vi "Mandelbrot_LabVIEW.vi"() -> ()   [LabVIEW 2020]
uses:
  <vilib>/Analysis/1siggen.llb/Ramp Pattern by Samples.vi
  5424d61b-997c-4bc6-ad91-23142d452257.vi
  acdee1ab-0b82-4047-983d-88c3d57dfc2c.vi
  <vilib>/Analysis/NI_AALBase.lvlib
panel:
  out "Device":string="Intel(R) Core(TM) i7-8700K"
  out "Current Frame":i32=223
  out "Time Elapsed":dbl=579.0 format="%#_3fs"
  out "Total Frames":i32=224
  out "Current Iters":i32=1500
  in  "Zoom Stop":dbl=1e-05 format="%#.9g"
  in  "Zoom Start":dbl=0.95 format="%#.9g"
  in  "Iters. Stop":i32=1500
  out "Time per Frame":dbl=3.86 format="%#_3ps"
  out "Current Zoom":dbl=1e-05
  in  "y":dbl=0.13182590420533 format="%#_17g"
  in  "x":dbl=-0.743643887037151 format="%#_18g"
  out "Mandelbrot Graph":i16[][](graph)
  in  "Iters. Start":i32=500
  in  "Resolution":i32=500
  # "Mandelbrot LabVIEW"
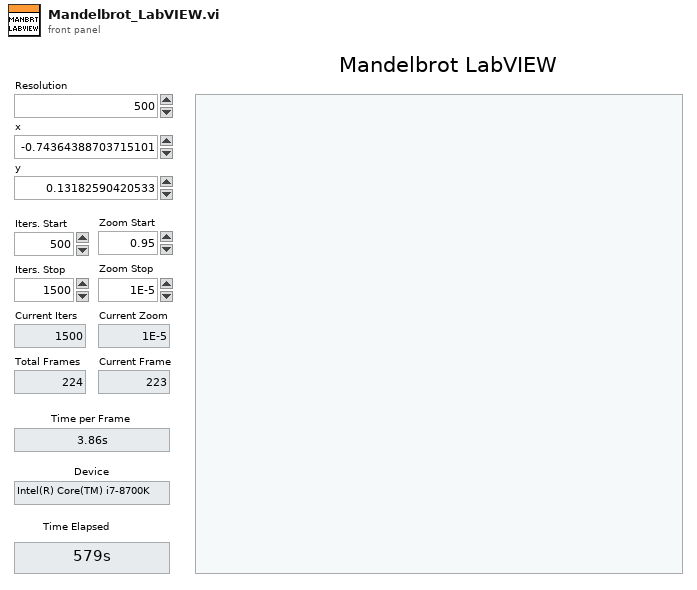
[diagram p1: front panel]
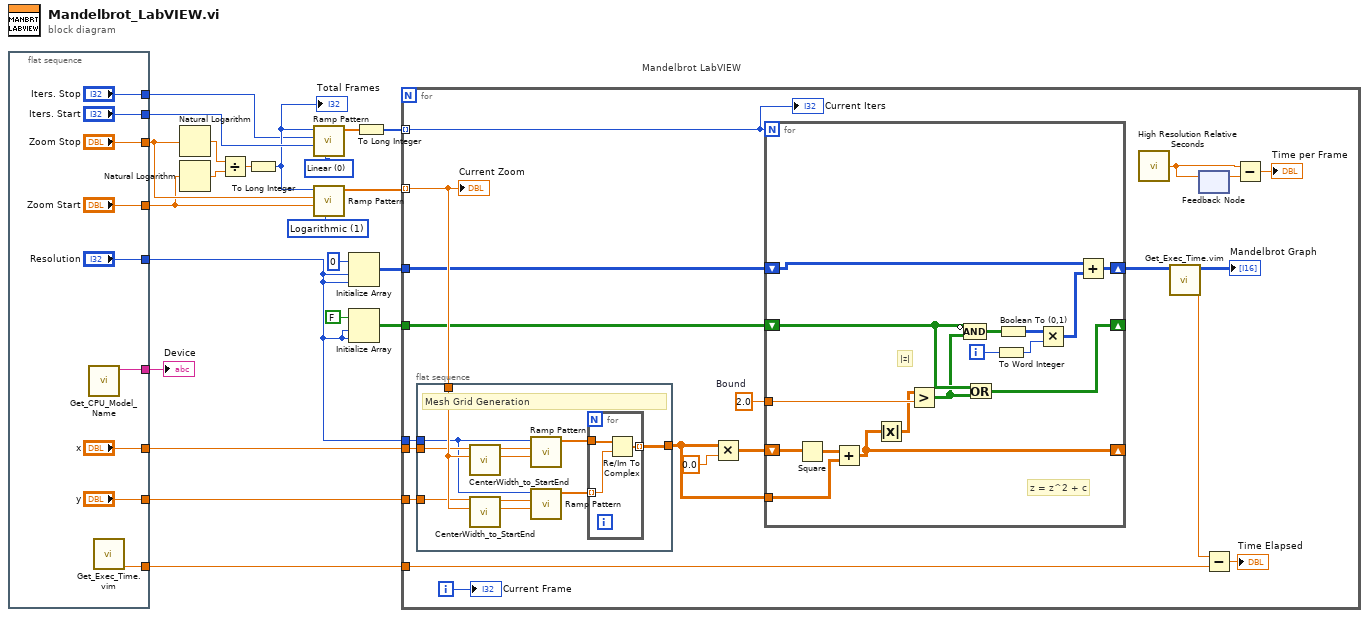
[diagram p0: block diagram]
diagram:
  w12 = u16 0 items=["Linear", "Logarithmic"] ("type")
  w11 = u16 1 items=["Linear", "Logarithmic"] ("type")
  # "Mandelbrot LabVIEW"
  n1 = flat-sequence {
    tunnel: ["Resolution"] -> w1
    tunnel: ["Iters. Start"] -> w17
    tunnel: ["Zoom Stop"] -> w14
    tunnel: ["Zoom Start"] -> w13
    tunnel: ["Iters. Stop"] -> w10
    tunnel: ["x"] -> w9
    tunnel: ["y"] -> w8
    tunnel: [w24] -> w7
    tunnel: [w23] -> w6
    frame #0 {
      n2 = call "Get_CPU_Model_Name.vi"() -> ("CPU Model"=w23:string)  [unwired: 11 in]
      n3 = call "Get_Exec_Time.vim"() -> ("T(n)"=w24:dbl)  [unwired: 7 in, 2 out]
    }
  }
  n4 = Natural Logarithm(1:w14) -> (0:w19:dbl)
  n5 = Natural Logarithm(1:w13) -> (0:w20:dbl)
  n6 = Divide(x=w19, y=w20) -> (x/y=w18:dbl)
  n7 = To Long Integer(number=w18) -> (32bit integer=w15:i32)
  "Total Frames" <- w15
  n8 = call-poly <vilib>:"Ramp Pattern.vi"("type"=w12, "start"=w17, "end"=w10, "samples"=w15) -> ("Ramp Pattern"=w16:dbl[])  [unwired: 6 in, 1 out]
  n9 = call-poly <vilib>:"Ramp Pattern.vi"("type"=w11, "start"=w13, "end"=w14, "samples"=w15) -> ("Ramp Pattern"=w21:dbl[])  [unwired: 6 in, 1 out]
  n10 = Initialize Array(i16 0 ("element"), w1, w1) -> (w4:i16[][])
  n11 = Initialize Array(FALSE, w1, w1) -> (w2:bool[][])
  n12 = To Long Integer(number=w16) -> (32bit integer=w22:i32[])
  n13 = for {
    tunnel: w4 -> [w46]
    tunnel: w2 -> [w34]
    tunnel: w22 -> [w48] mode=indexing
    tunnel: w21 -> [w47] mode=indexing
    tunnel: w7 -> [w40]
    tunnel: w9 -> [w36]
    tunnel: w8 -> [w35]
    tunnel: w1 -> [w33]
    i -> [w38]
    w43 = sgl 2.0  # Bound
    n14 = flat-sequence {
      tunnel: [w52] -> w51
      tunnel: w47 -> [w58]
      tunnel: w36 -> [w57]
      tunnel: w35 -> [w56]
      tunnel: w33 -> [w55]
      frame #0 {
        # "Mesh Grid Generation"
        n15 = call "CenterWidth_to_StartEnd.vi"("width"=w58, "Center"=w57) -> ("Start"=w61:dbl, "End"=w62:dbl)  [unwired: 8 in]
        n16 = call "CenterWidth_to_StartEnd.vi"("width"=w58, "Center"=w56) -> ("Start"=w59:dbl, "End"=w60:dbl)  [unwired: 8 in]
        n17 = call-poly <vilib>:"Ramp Pattern.vi"("start"=w61, "end"=w62, "samples"=w55) -> ("Ramp Pattern"=w54:dbl[])  [unwired: 7 in, 1 out]
        n18 = call-poly <vilib>:"Ramp Pattern.vi"("start"=w59, "end"=w60, "samples"=w55) -> ("Ramp Pattern"=w53:dbl[])  [unwired: 7 in, 1 out]
        n19 = for {
          tunnel: w54 -> [w65]
          tunnel: w53 -> [w64] mode=indexing
          tunnel: [w63] -> w52 mode=indexing
          n20 = Re/Im To Complex(1:w64, 2:w65) -> (0:w63:cdb[])
        }
      }
    }
    n21 = Multiply(x=w51, y=sgl 0.0 ("start")) -> (x*y=w45:cdb[][])
    n22 = for {
      N: w48 -> [_]
      shift-right: [w74] -> _
      shift-left: w45 -> [w77]
      tunnel: w51 -> [w79]
      shift-right: [w81] -> w32
      shift-left: w46 -> [w78]
      shift-right: [w80] -> _
      shift-left: w34 -> [w75]
      tunnel: w43 -> [w68]
      i -> [w69]
      # "|z|"
      # "z = z^2 + c"
      n23 = Square(x=w77) -> (x^2=w76:cdb[][])
      n24 = Add(x=w76, y=w79) -> (x+y=w74:cdb[][])
      n25 = Absolute Value(x=w74) -> (abs(x)=w67:dbl[][])
      n26 = Greater?(x=w67, y=w68) -> (0:w73:bool[][])
      n27 = Compound Arithmetic op=AND(invert w75, w73) -> (w72:bool[][])
      n28 = Or(x=w75, y=w73) -> (x .or. y?=w80:bool[][])
      n29 = To Word Integer(number=w69) -> (16bit integer=w66:i16)
      n30 = Boolean To (0,1)(Boolean=w72) -> (0, 1=w70:i16[][])
      n31 = Multiply(x=w70, y=w66) -> (x*y=w71:i16[][])
      n32 = Add(x=w78, y=w71) -> (x+y=w81:i16[][])
    }
    n33 = call <vilib>:"High Resolution Relative Seconds.vi"() -> ("relative seconds"=w42:dbl)
    n34 = call "Get_Exec_Time.vim"("error in (no error)"=w32) -> ("T(n)"=w41:dbl, "error out"=→"Mandelbrot Graph":i16[][])  [unwired: 6 in, 1 out]
    n35 = feedback #1() -> (w50:dbl)  [unwired: 1 in]
    n36 = feedback-in #1(w42) -> ()
    n37 = Subtract(x=w41, y=w40) -> (x-y=→"Time Elapsed":dbl)
    n38 = Subtract(x=w42, y=w50) -> (x-y=→"Time per Frame":dbl)
    "Current Zoom" <- w47
    "Current Iters" <- w48
    "Current Frame" <- w38
  }
  "Device" <- w6
